vi "test DOCTYPE Declaration (Case 7098).vi"(8 "error in (no error)":errorcluster, 11 "TestCase in":refnum<class "EasyXMLTest.lvclass">) -> (0 "error out":errorcluster, 3 "TestCase out":refnum<class "EasyXMLTest.lvclass">)   [LabVIEW 2013, in "EasyXMLTest.lvclass"]
doc: "Verify that error in is not overwritten"
uses:
  EasyXMLTest.lvclass
panel:
  out "Produced Data":variant
  out "Input Data":variant
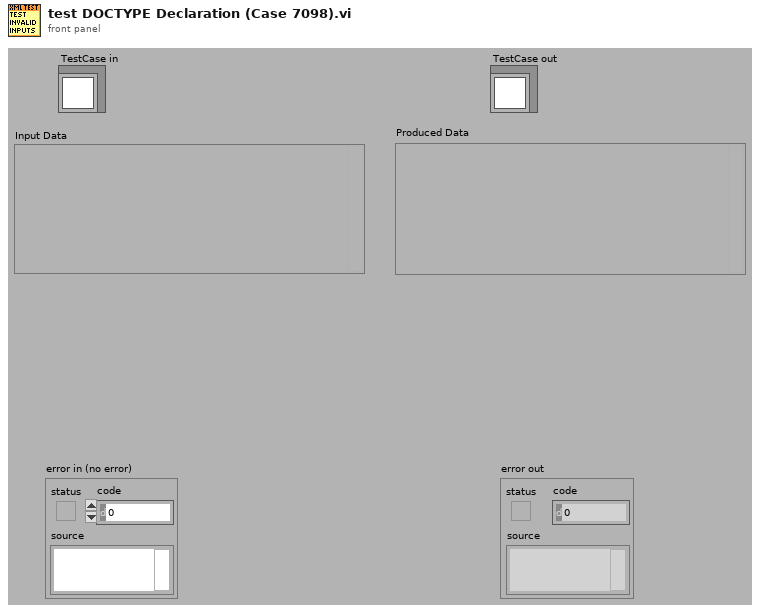
[diagram p1: front panel]
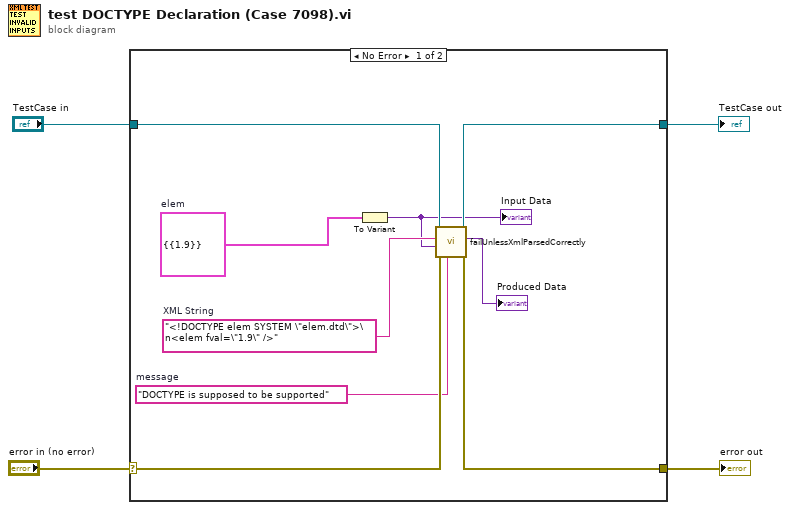
[diagram p0: block diagram]
diagram:
  n1 = case shown="No Error" "error in (no error)" {
    selector: "error in (no error)" -> [w8 w15]
    tunnel: [w7 w15] -> w2
    tunnel: [w12 w14] -> w1
    tunnel: "TestCase in" -> [w13 w14]
    frame No Error {
      w9 = cluster{"#attributes":cluster{"fval":dbl}} {"#attributes"={"fval"=1.9}}  # elem
      w10 = "<!DOCTYPE elem SYSTEM \"elem.dtd\">\n<elem fval=\"1.9\" />"  # XML String
      w6 = "DOCTYPE is supposed to be supported"  # message
      n2 = To Variant(anything=w9) -> (Variant=w5:variant)
      "Input Data" <- w5
      n3 = call "failUnlessXmlParsedCorrectly.vi"("message (\"\")"=w6, "error in"=w8, "Expected Data"=w5, "XML String"=w10, "reference in"=w13) -> ("error out"=w7:errorcluster, "Produced Data"=→"Produced Data":variant, "reference in"=w12:refnum<class "EasyXMLTest.lvclass">)  [unwired: 4 in]
    }
    frame Error {
    }
  }
  "error out" <- w2
  "TestCase out" <- w1
